vi "deploy absolute files.vi"(8 "error in (no error)":errorcluster, 11 "appended path":path) -> (0 "error out":errorcluster)   [LabVIEW 2014]
uses:
  absolute file spec.ctl
  <vilib>/Utility/xml.llb/Read From XML File(string).vi
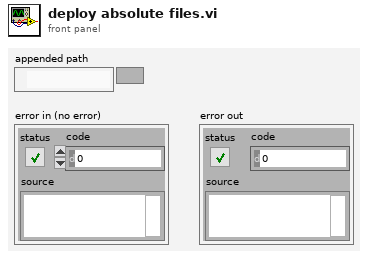
[diagram p1: front panel]
types:
  T1 = typedef "absolute file spec.ctl" = cluster{"name":string, "absolute path":path}
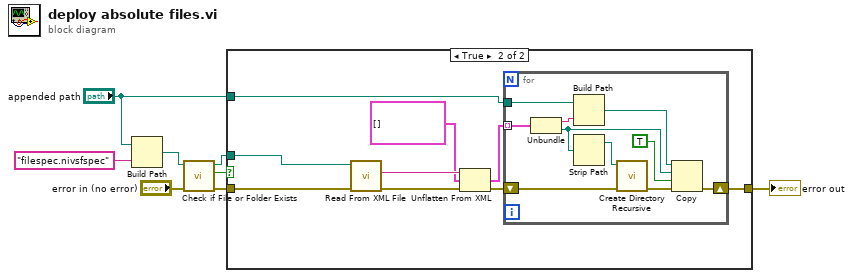
[diagram p0: block diagram]
diagram:
  n1 = Build Path(base path="appended path", name or relative path="filespec.nivsfspec") -> (appended path=w7:path)
  n2 = call <vilib>:"Check if File or Folder Exists.vi"("error in (no error)"="error in (no error)", "path"=w7) -> ("error out"=w3:errorcluster, "file or folder exists?"=w5:bool, "dup path"=w2:path)  [unwired: 7 in]
  n3 = case shown="True" w5 {
    tunnel: [w9 w12] -> w4
    tunnel: w3 -> [w9 w18]
    tunnel: w2 -> [_ w17]
    tunnel: "appended path" -> [_ w11]
    frame False {
    }
    frame True {
      n4 = call-poly <vilib>:"Read From XML File.vi"("error in (no error)"=w18, "XML File Path"=w17) -> ("error out"=w16:errorcluster, "XML Elements"=w15:string)  [unwired: 7 in, 1 out]
      n5 = Unflatten From XML(xml string=w15, type=T1[] [], error in (no error)=w16) -> (value=w10:T1[], error out=w13:errorcluster)
      n6 = for {
        shift-right: [w25] -> w12
        shift-left: w13 -> [w21]
        tunnel: w11 -> [w27]
        tunnel: w10 -> [w28] mode=indexing
        n7 = Unbundle(w28) -> ("name"=w26:string, "absolute path"=w22:path)
        n8 = Build Path(base path=w27, name or relative path=w26) -> (appended path=w23:path)
        n9 = Strip Path(path=w22) -> (stripped path=w20:path)  [unwired: 1 out]
        n10 = call <vilib>:"Create Directory Recursive.vi"("error in (no error)"=w21, "directory"=w20) -> ("error out"=w19:errorcluster)  [unwired: 3 in, 2 out]
        n11 = Copy(8:w19, 9:TRUE ("overwrite (F)"), 10:w22, 11:w23) -> (0:w25:errorcluster)  [unwired: 1 in, 2 out]
      }
    }
  }
  "error out" <- w4
